vi "InsertDataDsc.vi"(8 "error in (no error)":errorcluster caption="错误输入（无错误）", 10 "table":string, 11 "DscBoard":T1) -> (0 "error out":errorcluster caption="错误输出")   [LabVIEW 2014, in "DataBase.lvlib"]
uses:
  <vilib>/addons/database/Connection.llb/DB Tools Open Connec (String).vi
  DataBase.lvlib
  <vilib>/addons/database/NI_Database_API.lvlib
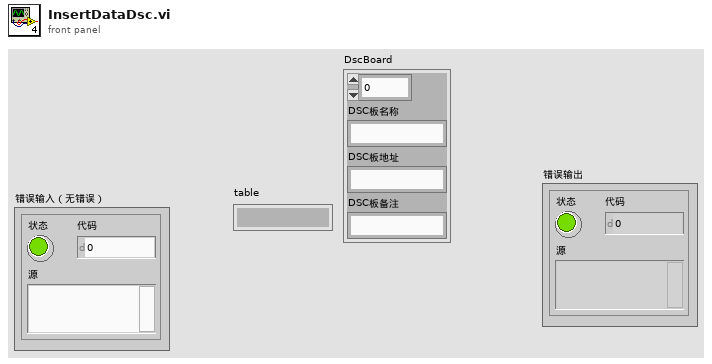
[diagram p1: front panel]
types:
  T1 = cluster{i32, "DSC板名称":string, "DSC板地址":string, "DSC板备注":string}
  T2 = typedef "NI_Database_API.lvlib/Conn ObjectReference.ctl" = refnum<k1>
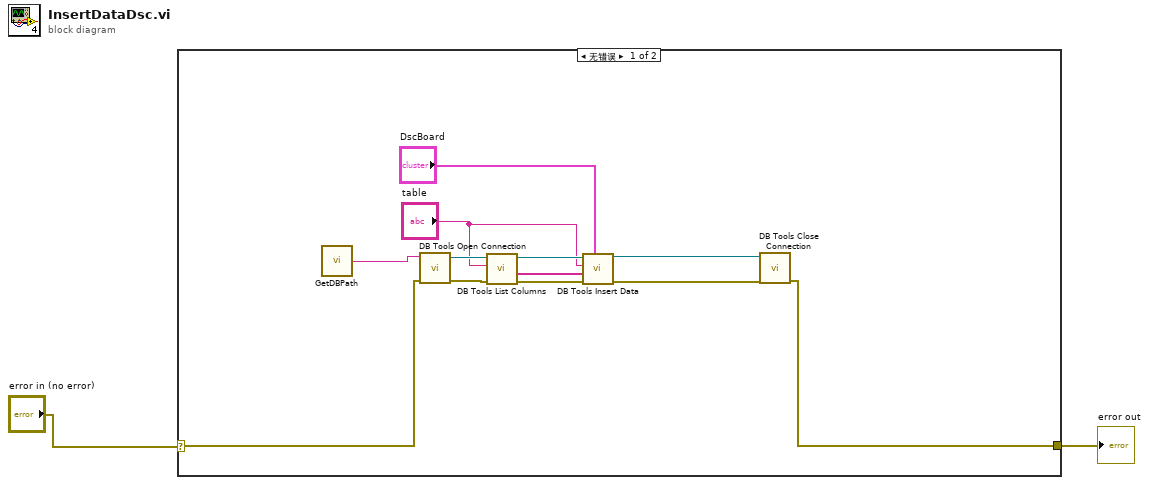
[diagram p0: block diagram]
diagram:
  n1 = case shown="无错误" "error in (no error)" {
    selector: "error in (no error)" -> [w11 w15]
    tunnel: [w7 w15] -> w1
    frame No Error {
      n2 = call "GetDBPath.vi"() -> ("Connection"=w14:string)  [unwired: 1 in]
      n3 = call-poly <vilib>:"DB Tools Open Connection.vi"("error in (no error)"=w11, "connection information"=w14) -> ("error out"=w10:errorcluster, "connection reference"=w13:T2)  [unwired: 6 in]
      n4 = call <vilib>:"DB Tools List Columns.vi"("error in (no error)"=w10, "table"="table", "connection reference"=w13) -> ("error out"=w9:errorcluster, "columns"=w4:string[], "connection reference out"=w12:T2)  [unwired: 1 in, 1 out]
      n5 = call <vilib>:"DB Tools Insert Data.vi"("data"="DscBoard", "error in (no error)"=w9, "columns"=w4, "table"="table", "connection reference"=w12) -> ("error out"=w8:errorcluster, "connection reference out"=w6:T2)  [unwired: 5 in]
      n6 = call <vilib>:"DB Tools Close Connection.vi"("error in (no error)"=w8, "connection reference"=w6) -> ("error out"=w7:errorcluster)  [unwired: 5 in]
    }
    frame Error {
    }
  }
  "error out" <- w1
